vi "FrequencyArrayToHz_SubVI.vi"(10 "Octave Range in":u32, 11 "Notes array in":dbl[](array[numeric])) -> (3 "Frequency array out":dbl[](array[numeric]))   [LabVIEW 2024]
doc: "This SubVI takes the array of notes in whole numbers and its octave range and returns an array of frequencies of said notes in the Western 12-note scale.\n\nIN: Notes array; Octave Range\nOUT: Freq. Array;"
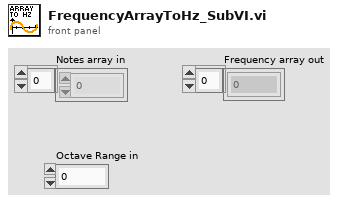
[diagram p1: front panel]
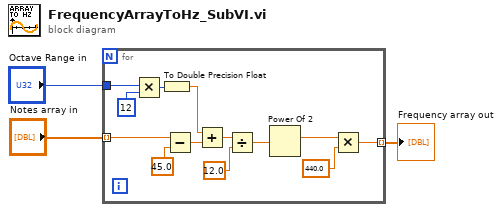
[diagram p0: block diagram]
diagram:
  n1 = for {
    tunnel: "Notes array in" -> [w16] mode=indexing
    tunnel: "Octave Range in" -> [w13]
    tunnel: [w6] -> w3 mode=indexing
    n2 = Multiply(x=w13, y=u32 12) -> (x*y=w11:u32)
    n3 = To Double Precision Float(number=w11) -> (double precision float=w10:dbl)
    n4 = Subtract(x=w16, y=45.0) -> (x-y=w14:dbl)
    n5 = Add(x=w10, y=w14) -> (x+y=w9:dbl)
    n6 = Divide(x=w9, y=12.0) -> (x/y=w7:dbl)
    n7 = Power Of 2(x=w7) -> (2^x=w5:dbl)
    n8 = Multiply(x=w5, y=440.0 ("x")) -> (x*y=w6:dbl)
  }
  "Frequency array out" <- w3
